vi "参数设置页.vi"() -> ()   [LabVIEW 2016, in "斯坦道通用流路CODmn.lvlib"]
uses:
  <vilib>/Plasmionique/MB Master/MB_Master/MB_Master.lvclass
  <vilib>/ptbypt/NI_PtbyPt.lvlib
panel:
  in  "手动模式":bool caption="手动模式(hd)"
  in  "简易流程周期设置":cluster{"switch button":bool, "设置按钮":bool}
  out "连接状态":bool
  in  "标样核查自动补测":bool caption="通讯连接"
  in  "跨度核查自动补测":bool caption="通讯连接"
  in  "零点核查自动补测":bool caption="通讯连接"
  in  "标样核查标液偏差":dbl caption="标样核查标液偏差："
  in  "跨度核查标液偏差":dbl caption="跨度核查标液偏差："
  in  "零点核查标液偏差":dbl caption="零点核查标液偏差："
  out "低量程上限":dbl caption="低量程上限："
  in  "简易流程路径":path=path "data/流程.xml"
  out "数据刷新时间":string
  in  "通讯连接":bool=TRUE
  out "MB table":enum32{"Serial", "TCP"}(tab)
  in  "请选择串口:":refnum<visa-resource-name>
  in  "IP":string="127.0.0.1"
  in  "PORT":string="1001"
  in  "通信方式选择":enum16{"串口", "TCP"}(ring)
  in  "盐度自动补偿：":bool
  out "盐度补偿值":dbl caption="盐度补偿值："
  in  "刷新":bool
  in  "测量模式":T1(ring)
  in  "参数下拉列表":u16(ring)
  in  "量程下拉列表":enum16{"低量程", "高量程"}(ring)
  in  "测试流程路径":path=path "data/流程.xml"
  in  "标样核查量程模式":T2 caption="标样核查："
  in  "加标回收量程模式":T2 caption="加标回收："
  in  "跨度核查量程模式":T2 caption="跨度核查："
  in  "零点核查量程模式":T2 caption="零点核查："
  in  "水样测试量程模式":T2 caption="水样测试："
  out "稀释度":dbl caption="稀释度："
  out "阈值（高->低）":dbl caption="阈值（高->低）："
  out "阈值（低->高）":dbl caption="阈值（低->高）："
  out "量程下限":dbl caption="量程下限："
  out "高量程上限":dbl caption="高量程上限："
  out "检出限":dbl caption="检出限："
  out "曲线截距":dbl caption="曲线截距：" format="%#.6f"
  out "曲线斜率":dbl caption="曲线斜率：" format="%#.6f"
  out "二次多项式系数":dbl caption="二次多项式系数：" format="%#.6f"
  out "消解时长":dbl caption="消解时长："
  out "消解温度":dbl caption="消解温度："
  out "测量精度":u16 caption="测量精度："
  in  "标样核查标液浓度":dbl caption="标样核查标液浓度："
  in  "跨度核查标液浓度":dbl caption="跨度核查标液浓度："
  in  "零点核查标液浓度":dbl caption="零点核查标液浓度："
  in  "跨度值":dbl caption="跨度值："
  # "日质控设置"
  # "关键参数"
  # "连接设置"
  # "mg/L"
  # "mg/L"
  # "mg/L"
  # "mg/L"
  # "±"
  # "%"
  # "%"
  # "流程设置"
  # "简易流程周期设置"
  # "自动测试量程设置"
  # "设置："
  # "mg/L"
  # "ppt"
  # "mg/L"
  # "mg/L"
  # "mg/L"
  # "mg/L"
  # "mg/L"
  # "min"
  # "℃"
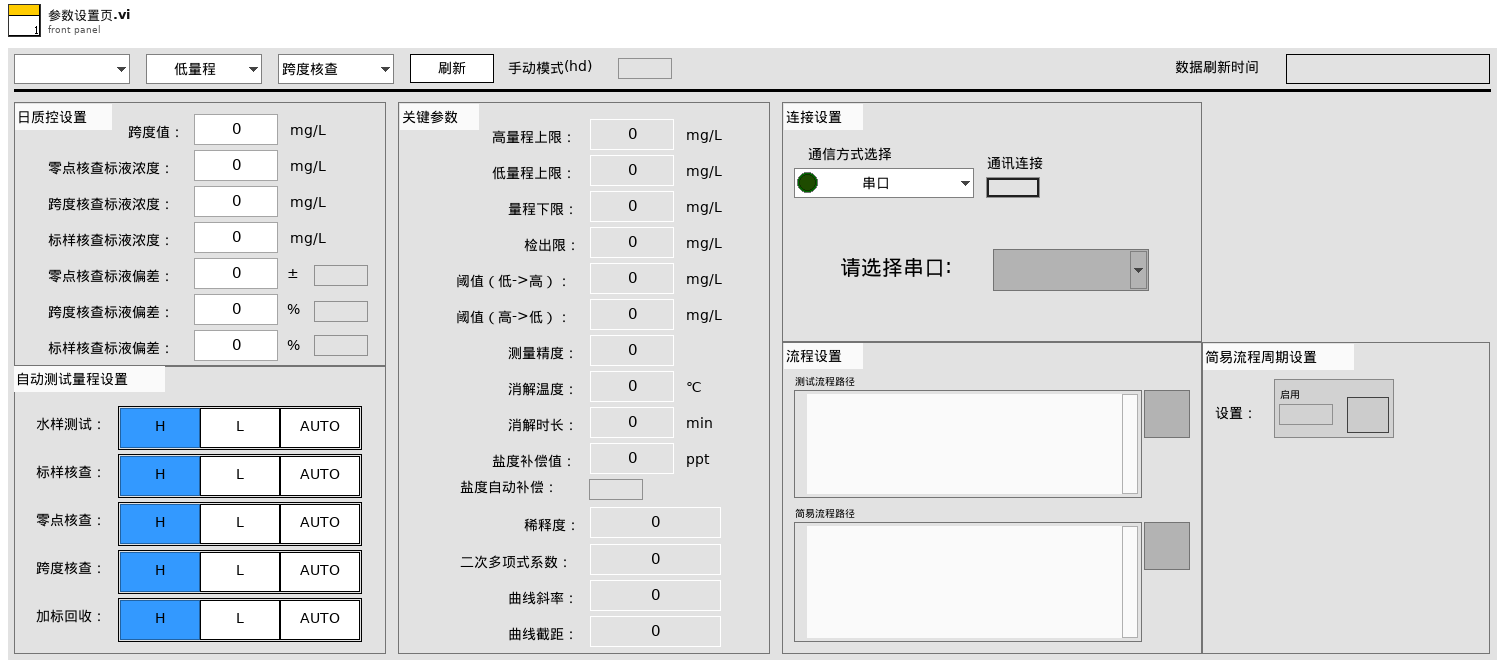
[diagram p1: front panel]
types:
  T1 = enum16{"跨度核查", "水样测量", "零点核查", "标样核查", "加标回收", "平行样测试", "空白校准", "标样校准", "空白测试"}
  T2 = typedef "斯坦道通用流路CODmn.lvlib/量程模式.ctl" = enum32{"H", "L", "AUTO"}
  T3 = typedef "Cleaning cycle.lvclass/周期项.ctl" = cluster{"时":i32, "分":i32, "频次":string, "id":i32, "参数":string, "simpleflowid":i32, "简易流程名称":string}
  T4 = cluster{"系统时间":timestamp, "工作状态":u16, "测量模式":enum16{"待机", "连续模式", "周期模式", "定点模式", "受控模式", "手动模式"}, "告警代码":u16, "故障代码":u16, "日志代码":u16, "软件版本":u16, "F0":sgl, "F1":sgl, "F2":sgl, "F3":sgl, "T":sgl, "H":sgl, "id":u16, "flowid":u16, "量程":u16, "总磷控温温度1":sgl, "营养盐控温温度2":sgl, "ADC":sgl, "结果值":sgl, "运行时间":u16, "步骤详情":string, "步骤流程":string}
  T5 = typedef "LVStringsAndValuesArrayTypeDef_U16.ctl" = cluster{"String":string, "Value":u16}[]
  T6 = enum8{"Enabled", "Disabled", "Disabled and Grayed Out"}
  T7 = cluster{"测量精度":u16, "检出限":dbl, "上限":dbl, "下限":dbl, "阈值（低->高）":dbl, "阈值（高->低）":dbl, "稀释度":dbl}
  T8 = typedef "操作日志字段定义.ctl" = cluster{"时间":timestamp, "参数":string, "日志信息":string, "流程参数":string}
  T9 = typedef "SingleStepTestV3.lvlib/SingleStepTestV3.lvclass/仪器版本.ctl" = enum16{"V3.1版", "V4版", "V3版", "V4.2版"}
  T10 = typedef "斯坦道通用流路CODmn.lvlib/V3.1版外设参数.ctl" = cluster{"泵类型":u8, "进样速度":u32, "出样速度":u32, "泵阀量":u8, "阀方向":u8, "光谱仪类型":u8, "光谱采样次数":u8, "氙灯次数":u8, "B":u16, "C":u16, "D":u16, "E":u16, "B_COD":u16, "C_COD":u16, "D_COD":u16, "E_COD":u16, "G":u16, "M":u16, "N":u16, "氨氮注射泵控温下限":sgl, "氨氮注射泵控温上限":sgl, "总氮注射泵控温下限":sgl, "总氮注射泵控温上限":sgl, "消解温度下限":sgl, "消解温度上限":sgl, "加热10s限值":sgl, "KP":sgl, "KI":sgl, "KD":sgl, "高温高压阀开阀温度":sgl, "总氮x公式0":u8, "总氮x公式1":sgl, "总氮x公式2":sgl, "总磷浊度稀释系数":sgl, "总磷浊度补偿权重1":sgl, "总磷浊度补偿权重2":sgl, "盐度系数":sgl, "氨氮补偿系数1":sgl, "氨氮补偿系数2":sgl}
  T11 = typedef "斯坦道通用流路CODmn.lvlib/V4版外设参数.ctl" = cluster{"泵类型":u8, "注射泵正常速度":u32, "注射泵慢速":u32, "阀型号":u8, "res":u8, "光谱仪类型":u8, "光谱采样次数":u8, "氙灯次数":u8, "B":u16, "C":u16, "D":u16, "E":u16, "B_COD":u16, "C_COD":u16, "D_COD":u16, "E_COD":u16, "G":u16, "M":u16, "N":u16, "降温下限":sgl, "降温上限":sgl, "恒温温度下限":sgl, "恒温温度上限":sgl, "消解温度下限":sgl, "消解温度上限":sgl, "加热10s限值":sgl, "KP":sgl, "KI":sgl, "KD":sgl, "高温高压阀开阀温度":sgl, "总氮x公式0":u8, "总氮x公式1":sgl, "总氮x公式2":sgl, "总磷浊度稀释系数":sgl, "总磷浊度补偿权重1":sgl, "总磷浊度补偿权重2":sgl, "盐度系数":sgl, "氨氮补偿系数1":sgl, "氨氮补偿系数2":sgl, "缺试剂传感器阈值":u16}
  T12 = typedef "斯坦道通用流路CODmn.lvlib/V4.2版外设参数.ctl" = cluster{"工作模式":u16, "泵类型":u16, "阀型号":u16, "注射泵进样速度":u16, "注射泵出样速度":u16, "注射泵滴定速度":u16, "res":u16, "注射泵慢速":u16, "光谱仪类型":u16, "光谱采样次数":u16, "氙灯次数":u16, "B":u16, "C":u16, "D":u16, "E":u16, "B_COD":u16, "C_COD":u16, "D_COD":u16, "E_COD":u16, "G":u16, "M":u16, "N":u16, "温度校准参数":sgl, "降温温度":sgl, "恒温温度":sgl, "消解温度":sgl, "高温高压阀开阀温度":sgl, "加热超时时间":sgl, "KP":sgl, "KI":sgl, "KD":sgl, "消解PID积分上限":sgl, "恒温PID积分上限":sgl, "PID积分下限":sgl, "缺试剂传感器阈值":u16, "滴定延时":u16, "滴定斜率阈值":sgl, "总氮x公式0":u16, "总氮x公式1":sgl, "总氮x公式2":sgl, "总磷浊度稀释系数":sgl, "总磷浊度补偿权重1":sgl, "总磷浊度补偿权重2":sgl, "盐度系数":sgl, "氨氮补偿系数1":sgl, "氨氮补偿系数2":sgl}
  T13 = typedef "斯坦道通用流路CODmn.lvlib/V3版外设参数.ctl" = cluster{"泵类型":u8, "进样速度":u32, "出样速度":u32, "泵阀量":u8, "光谱仪类型":u8, "光谱采样次数":u8, "氙灯次数":u8, "B":u16, "C":u16, "D":u16, "E":u16, "B_COD":u16, "C_COD":u16, "D_COD":u16, "E_COD":u16, "G":u16, "M":u16, "N":u16, "氨氮注射泵控温下限":sgl, "氨氮注射泵控温上限":sgl, "总氮注射泵控温下限":sgl, "总氮注射泵控温上限":sgl, "消解温度下限":sgl, "消解温度上限":sgl, "加热10s限值":sgl, "高温高压阀开阀温度":sgl, "总氮x公式0":u8, "总氮x公式1":sgl, "总氮x公式2":sgl, "总磷浊度稀释系数":sgl, "总磷浊度补偿权重1":sgl, "总磷浊度补偿权重2":sgl, "盐度系数":sgl, "氨氮补偿系数1":sgl, "氨氮补偿系数2":sgl}
  T14 = cluster{"水样测试量程模式":T2, "零点核查量程模式":T2, "跨度核查量程模式":T2, "加标回收量程模式":T2, "标样核查量程模式":T2}
  T15 = cluster{"总磷":dbl, "总氮":dbl, "氨氮":dbl, "磷酸盐":dbl, "硝氮":dbl, "亚硝氮":dbl, "硅酸盐":dbl, "硫化物":dbl, "COD":dbl, "氟化物":dbl, "CODMn":dbl}
  T16 = cluster{"总磷跨度值":dbl, "总磷零点标准液浓度":dbl, "总磷跨度标准液浓度":dbl, "总磷标准液标准浓度":dbl, "总氮跨度值":dbl, "总氮零点标准液浓度":dbl, "总氮跨度标准液浓度":dbl, "总氮标准液标准浓度":dbl, "COD跨度值":dbl, "COD零点标准液浓度":dbl, "COD跨度标准液浓度":dbl, "COD标准液标准浓度":dbl, "氨氮跨度值":dbl, "氨氮零点标准液浓度":dbl, "氨氮跨度标准液浓度":dbl, "氨氮标准液标准浓度":dbl, "磷酸盐跨度值":dbl, "磷酸盐零点标准液浓度":dbl, "磷酸盐跨度标准液浓度":dbl, "磷酸盐标准液标准浓度":dbl, "硝氮跨度值":dbl, "硝氮零点标准液浓度":dbl, "硝氮跨度标准液浓度":dbl, "硝氮标准液标准浓度":dbl, "亚硝氮跨度值":dbl, "亚硝氮零点标准液浓度":dbl, "亚硝氮跨度标准液浓度":dbl, "亚硝氮标准液标准浓度":dbl, "硫化物跨度值":dbl, "硫化物零点标准液浓度":dbl, "硫化物跨度标准液浓度":dbl, "硫化物标准液标准浓度":dbl, "硅酸盐跨度值":dbl, "硅酸盐零点标准液浓度":dbl, "硅酸盐跨度标准液浓度":dbl, "硅酸盐标准液标准浓度":dbl, "总磷零点标准液偏差":dbl, "总磷跨度标准液偏差":dbl, "总磷标准液标准偏差":dbl, "总氮零点标准液偏差":dbl, "总氮跨度标准液偏差":dbl, "总氮标准液标准偏差":dbl, "COD零点标准液偏差":dbl, "COD跨度标准液偏差":dbl, "COD标准液标准偏差":dbl, "氨氮零点标准液偏差":dbl, "氨氮跨度标准液偏差":dbl, "氨氮标准液标准偏差":dbl, "磷酸盐零点标准液偏差":dbl, "磷酸盐跨度标准液偏差":dbl, "磷酸盐标准液标准偏差":dbl, "硝氮零点标准液偏差":dbl, "硝氮跨度标准液偏差":dbl, "硝氮标准液标准偏差":dbl, "亚硝氮零点标准液偏差":dbl, "亚硝氮跨度标准液偏差":dbl, "亚硝氮标准液标准偏差":dbl, "硫化物零点标准液偏差":dbl, "硫化物跨度标准液偏差":dbl, "硫化物标准液标准偏差":dbl, "硅酸盐零点标准液偏差":dbl, "硅酸盐跨度标准液偏差":dbl, "硅酸盐标准液标准偏差":dbl, "氟化物跨度值":dbl, "氟化物零点标准液浓度":dbl, "氟化物跨度标准液浓度":dbl, "氟化物标准液标准浓度":dbl, "氟化物零点标准液偏差":dbl, "氟化物跨度标准液偏差":dbl, "氟化物标准液标准偏差":dbl, "CODMn跨度值":dbl, "CODMn零点标准液浓度":dbl, "CODMn跨度标准液浓度":dbl, "CODMn标准液标准浓度":dbl, "CODMn零点标准液偏差":dbl, "CODMn跨度标准液偏差":dbl, "CODMn标准液标准偏差":dbl}
  T17 = cluster{"水样测试量程模式":enum16{"H", "L", "AUTO"}, "空白核查量程模式":enum16{"H", "L", "AUTO"}, "跨度核查量程模式":enum16{"H", "L", "AUTO"}, "加标回收量程模式":enum16{"H", "L", "AUTO"}, "标样核查量程模式":enum16{"H", "L", "AUTO"}}
  T18 = cluster{"水样测试量程模式":u16, "空白核查量程模式":u16, "跨度核查量程模式":u16, "加标回收量程模式":u16, "标样核查量程模式":u16}
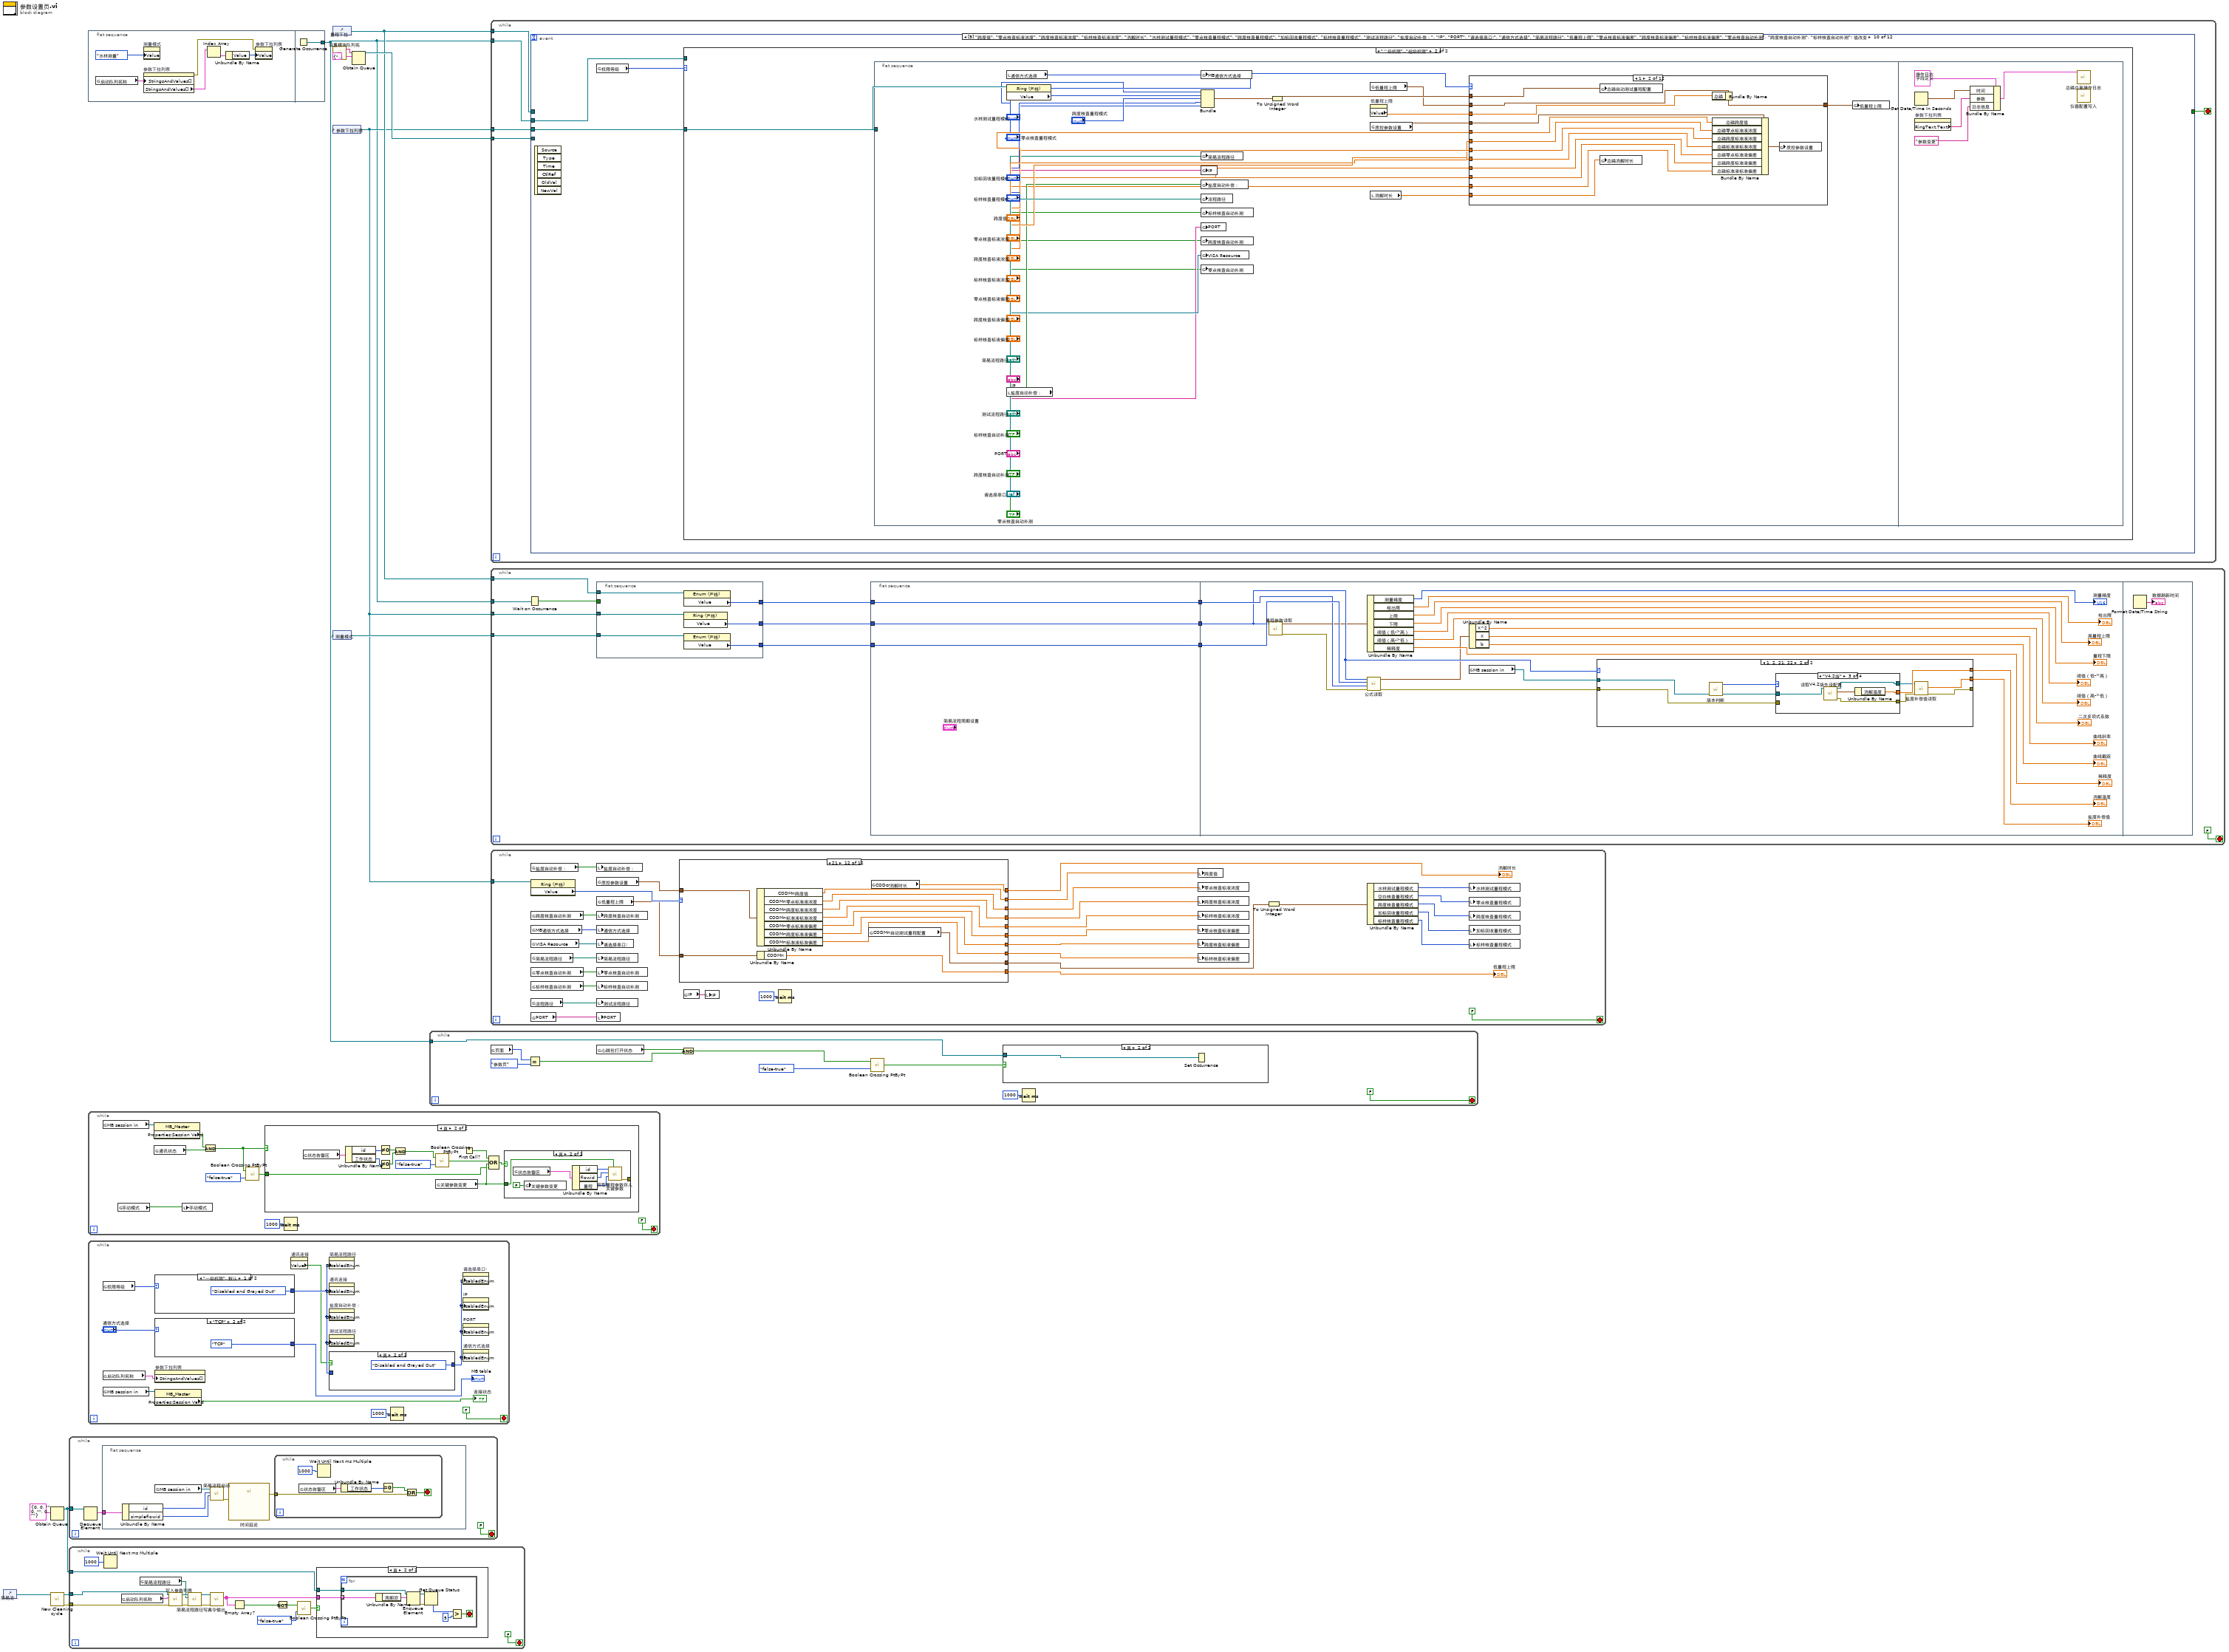
[diagram p0: block diagram]
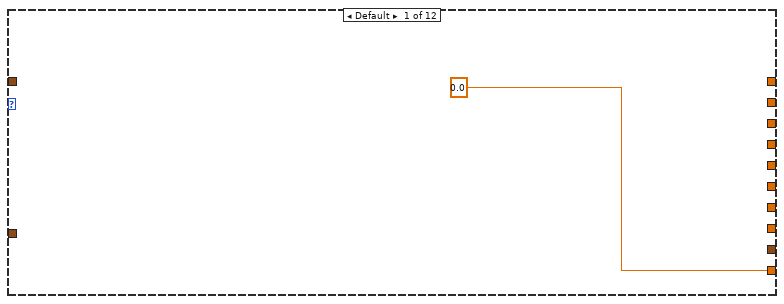
[diagram p6: hidden frame]
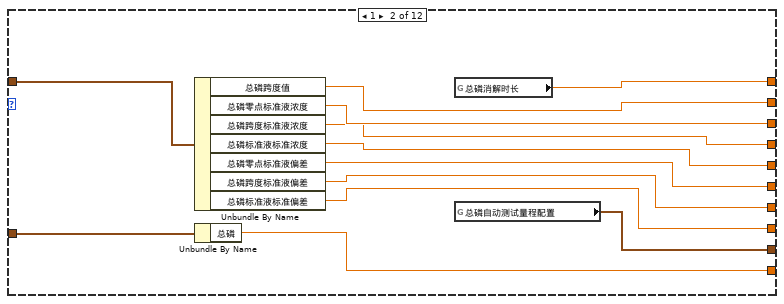
[diagram p7: hidden frame]
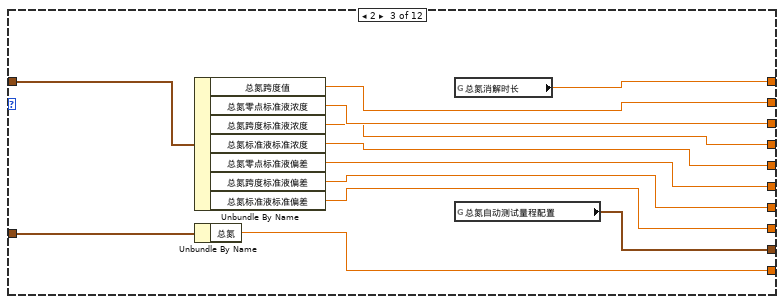
[diagram p8: hidden frame]
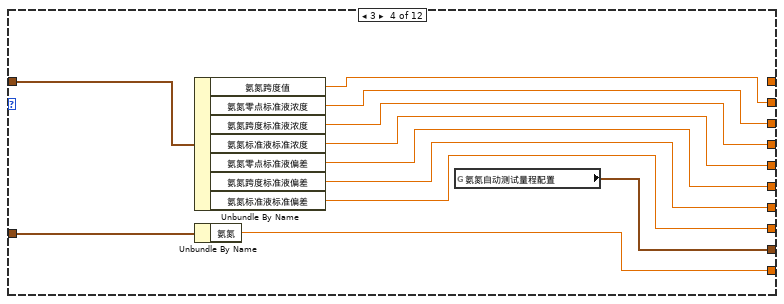
[diagram p9: hidden frame]
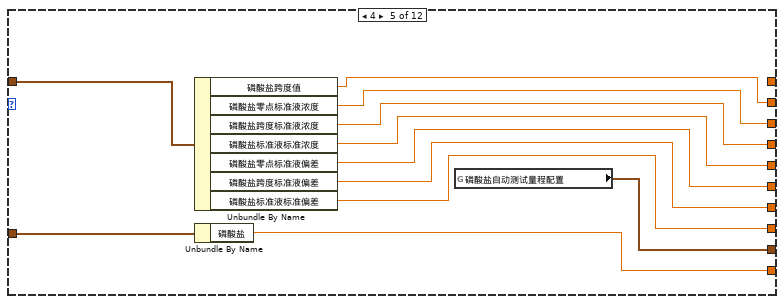
[diagram p10: hidden frame]
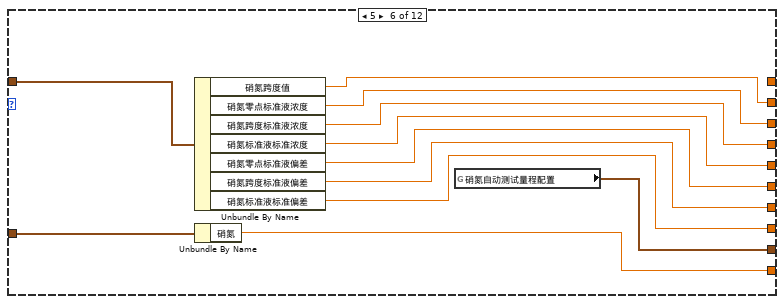
[diagram p11: hidden frame]
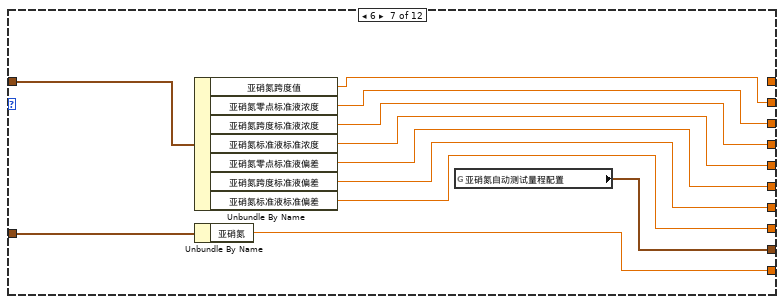
[diagram p12: hidden frame]
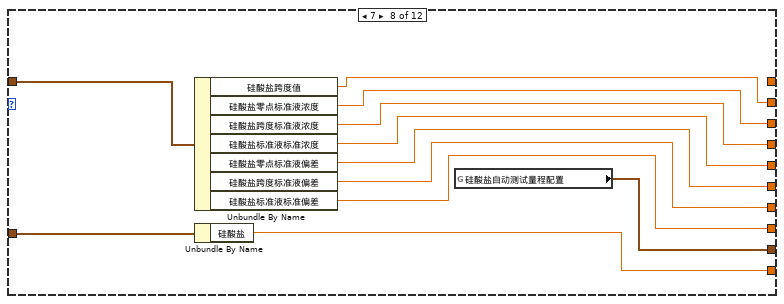
[diagram p13: hidden frame]
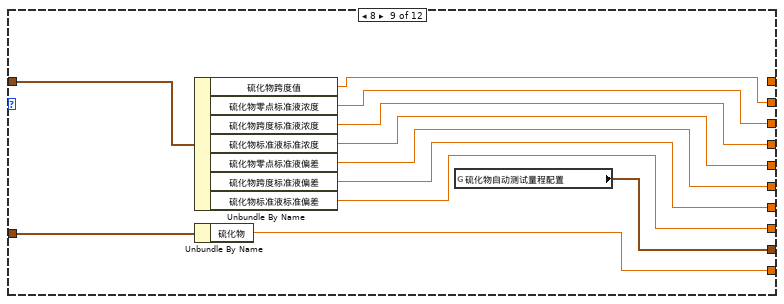
[diagram p14: hidden frame]
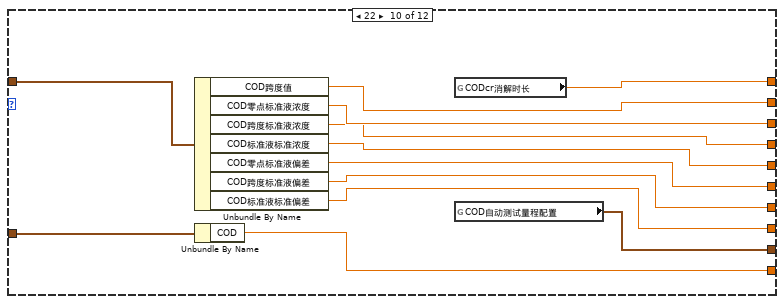
[diagram p15: hidden frame]
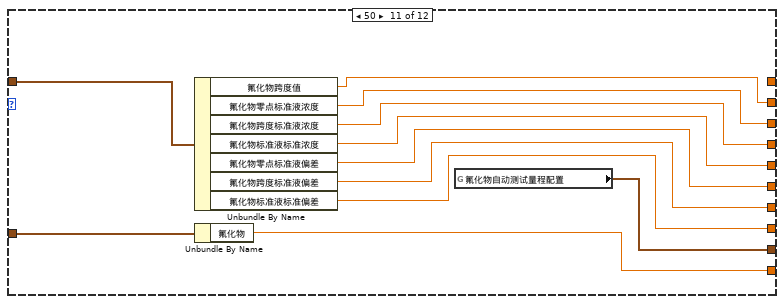
[diagram p16: hidden frame]
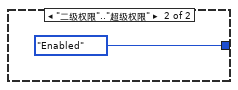
[diagram p17: hidden frame]
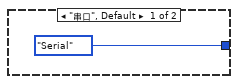
[diagram p18: hidden frame]
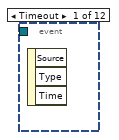
[diagram p20: hidden frame]
diagram:
  n1 = control-ref of="简易流程周期设置"() -> (w3:refnum<vi>)
  n2 = Obtain Queue(element data type=T3 {"时"=0, "分"=0, "频次"="", "id"=0, "参数"="", "simpleflowid"=0, "简易流程名称"=""} ("周期项")) -> (queue out=w1:refnum<queue>)  [unwired: 4 in, 2 out]
  n3 = call "New Cleaning cycle.vi"("Reference"=w3) -> ("error out"=w4:errorcluster, "Cleaningcycle out"=w5:refnum<class "Cleaning cycle.lvclass">)  [unwired: 9 in]
  n4 = while {
    tunnel: w1 -> [w15]
    stop <- FALSE stop-if-true
    n5 = Dequeue Element(queue=w15) -> (element=w14:T3)  [unwired: 2 in, 3 out]
    n6 = flat-sequence {
      tunnel: w14 -> [w20]
      frame #0 {
        n7 = Unbundle By Name(w20) -> ("id"=w18:i32, "simpleflowid"=w19:i32)
        n8 = global read "VAR总磷总氮全局变量.vi" "MB session in"() -> (w21:refnum<class "MB_Master.lvclass">)
        n9 = call "简易流程启动.vi"("简易流程"=w19, "参数Id"=w18, "MB session in"=w21) -> ("error out"=w17:errorcluster)  [unwired: 7 in, 1 out]
        n10 = call "时间延迟"("error in (no error)"=w17) -> ("error out"=w16:errorcluster)  [unwired: 10 in]
        n11 = while {
          tunnel: w16 -> [w23]
          stop <- w22 stop-if-true
          n12 = global read "VAR总磷总氮全局变量.vi" "状态告警区"() -> (w26:T4)
          n13 = Wait Until Next ms Multiple(millisecond multiple=u32 1000 ("毫秒倍数")) -> ()  [unwired: 1 out]
          n14 = Unbundle By Name(w26) -> ("工作状态"=w25:u16)
          n15 = Equal To 0?(x=w25) -> (x = 0?=w24:bool)
          n16 = Or(x=w24, y=w23) -> (x .or. y?=w22:bool)
        }
      }
    }
  }
  n17 = while {
    tunnel: w5 -> [w43]
    tunnel: w4 -> [w42]
    tunnel: w1 -> [w29]
    stop <- FALSE stop-if-true
    n18 = Wait Until Next ms Multiple(millisecond multiple=u32 1000 ("毫秒倍数")) -> ()  [unwired: 1 out]
    n19 = global read "model config var.vi" "启动队列名称"() -> (w39:cluster{"String":string, "Value":u16}[])
    n20 = global read "总磷总氮断电保存全局变量.vi" "简易流程路径"() -> (w38:path)
    n21 = call "写入参数列表.vi"("error in (no error)"=w42, "参数列表"=w39, "Cleaningcycle 输入"=w43) -> ("error out"=w41:errorcluster, "Cleaningcycle 输出"=w40:refnum<class "Cleaning cycle.lvclass">)  [unwired: 7 in]
    n22 = call "简易流程路径写入.vi"("error in (no error)"=w41, "简易流程路径"=w38, "Cleaningcycle 输入"=w40) -> ("error out"=w36:errorcluster, "Cleaningcycle 输出"=w37:refnum<class "Cleaning cycle.lvclass">)  [unwired: 7 in]
    n23 = call "命令输出.vi"("error in (no error)"=w36, "Cleaningcycle 输入"=w37) -> ("命令"=w31:cluster{"触发":bool, "周期项":T3}[])  [unwired: 7 in, 2 out]
    n24 = Empty Array?(array=w31) -> (empty?=w35:bool)
    n25 = Not(x=w35) -> (.not. x?=w34:bool)
    n26 = call <vilib>:"Boolean Crossing PtByPt.vi"("direction"=enum16{"either", "false-true", "true-false"}."false-true", "input"=w34) -> ("crossing"=w32:bool)  [unwired: 1 in]
    n27 = case shown="真" w32 {
      tunnel: w31 -> [_ w45]
      tunnel: w29 -> [_ w44]
      frame False {
      }
      frame True {
        n28 = for {
          tunnel: w45 -> [w53] mode=indexing
          tunnel: w44 -> [w51]
          stop <- w46 stop-if-true
          n29 = Unbundle By Name(w53) -> ("周期项"=w52:T3)
          n30 = Enqueue Element(queue=w51, element=w52) -> (queue out=w50:refnum<queue>, error out=w49:errorcluster)  [unwired: 2 in, 1 out]
          n31 = Get Queue Status(queue=w50, error in (no error)=w49) -> (# elements in queue=w48:i32)  [unwired: 1 in, 7 out]
          n32 = Greater?(x=w48, y=5) -> (0:w46:bool)
        }
      }
    }
  }
  n33 = flat-sequence {
    tunnel: [w60] -> w6
    frame #0 {
      n34 = global read "model config var.vi" "启动队列名称"() -> (w55:cluster{"String":string, "Value":u16}[])
      n35 = property on="测量模式" class="Enum (严格)"("Value"=T1."水样测量" ("测量模式")) -> ()  [unwired: 2 in, 2 out]
      n36 = property on="参数下拉列表" class="Ring (严格)"("StringsAndValues[]"=w55) -> (error out=w58:errorcluster, "StringsAndValues[]"=w56:T5)  [unwired: 2 in, 1 out]
      n37 = Index Array(array=w56) -> (element=w57:cluster{"String":string, "Value":u16})  [unwired: 1 in]
      n38 = Unbundle By Name(w57) -> ("Value"=w59:u16)
      n39 = property on="参数下拉列表" class="Ring (严格)"(error in=w58, "Value"=w59) -> ()  [unwired: 1 in, 2 out]
    }
    frame #1 {
      n40 = Generate Occurrence() -> (w60:refnum<k4>)
    }
  }
  n41 = while {
    stop <- FALSE stop-if-true
    n42 = global read "VAR总磷总氮全局变量.vi" "MB session in"() -> (w66:refnum<class "MB_Master.lvclass">)
    n43 = global read "VAR总磷总氮全局变量.vi" "手动模式"() -> (w61:bool)
    n44 = property class="MB_Master"(reference=w66) -> ("Properties:Session Valid"=w65:bool)  [unwired: 1 in, 2 out]
    n45 = global read "VAR总磷总氮全局变量.vi" "通讯状态"() -> (w68:bool)
    n46 = local write "手动模式"(w61) -> ()
    n47 = And(x=w65, y=w68) -> (x .and. y?=w63:bool)
    n48 = call <vilib>:"Boolean Crossing PtByPt.vi"("direction"=enum16{"either", "false-true", "true-false"}."false-true", "input"=w63) -> ("crossing"=w62:bool)  [unwired: 1 in]
    n49 = case shown="真" w63 {
      tunnel: w62 -> [_ w71]
      frame False {
      }
      frame True {
        n50 = global read "VAR总磷总氮全局变量.vi" "状态告警区"() -> (w81:T4)
        n51 = Unbundle By Name(w81) -> ("id"=w75:u16, "工作状态"=w80:u16)
        n52 = Not Equal To 0?(x=w75) -> (x != 0?=w76:bool)
        n53 = Not Equal To 0?(x=w80) -> (x != 0?=w77:bool)
        n54 = And(x=w76, y=w77) -> (x .and. y?=w78:bool)
        n55 = call <vilib>:"Boolean Crossing PtByPt.vi"("direction"=enum16{"either", "false-true", "true-false"}."false-true", "input"=w78) -> ("crossing"=w74:bool)  [unwired: 1 in]
        n56 = global read "VAR总磷总氮全局变量.vi" "关键参数变更"() -> (w72:bool)
        n57 = First Call?() -> (First Call?: T/F=w70:bool)
        n58 = Compound Arithmetic op=OR ("复合运算")(w70, w74, w72, w71) -> (w73:bool)
        n59 = case shown="真" w73 {
          tunnel: [_ w88] -> _
          tunnel: w72 -> [_ w83]
          frame False {
          }
          frame True {
            n60 = global read "VAR总磷总氮全局变量.vi" "状态告警区"() -> (w87:T4)
            n61 = global write "VAR总磷总氮全局变量.vi" "关键参数变更"(FALSE ("关键参数变更")) -> ()
            n62 = Unbundle By Name(w87) -> ("id"=w86:u16, "flowid"=w85:u16, "量程"=w84:u16)
            n63 = call "获取量程参数存入关键参数.vi"("关键参数变更"=w83, "量程"=w84, "flowid"=w85, "id"=w86) -> ("error out"=w88:errorcluster)  [unwired: 7 in]
          }
        }
      }
    }
    n64 = Wait (ms)(milliseconds to wait=u32 1000 ("等待时间（毫秒）")) -> ()  [unwired: 1 out]
  }
  n65 = while {
    stop <- FALSE stop-if-true
    n66 = global read "VAR总磷总氮全局变量.vi" "权限等级"() -> (w93:enum16{"一级权限", "二级权限", "三级权限", "超级权限"})
    n67 = global read "model config var.vi" "启动队列名称"() -> (w91:cluster{"String":string, "Value":u16}[])
    n68 = global read "VAR总磷总氮全局变量.vi" "MB session in"() -> (w98:refnum<class "MB_Master.lvclass">)
    n69 = case shown="\"一级权限\", 默认" w93 {
      tunnel: [T6."Disabled and Grayed Out" ("禁用") T6."Enabled" ("禁用")] -> w92
      frame "一级权限", Default {
      }
      frame "二级权限".."超级权限" {
      }
    }
    n70 = case shown="\"TCP\"" "通信方式选择" {
      tunnel: [enum32{"Serial", "TCP"}."Serial" ("MB table") enum32{"Serial", "TCP"}."TCP" ("MB table")] -> w95
      frame "串口", Default {
      }
      frame "TCP" {
      }
    }
    "MB table" <- w95
    n71 = property on="参数下拉列表" class="Ring (严格)"("StringsAndValues[]"=w91) -> ()  [unwired: 2 in, 2 out]
    n72 = property class="MB_Master"(reference=w98) -> ("Properties:Session Valid"=→"连接状态":bool)  [unwired: 1 in, 2 out]
    n73 = property on="通讯连接" class="Bool (严格)"() -> ("Value"=w89:bool)  [unwired: 2 in, 2 out]
    n74 = property on="简易流程路径" class="Path"("DisabledEnum"=w92) -> ()  [unwired: 2 in, 2 out]
    n75 = property on="通讯连接" class="Bool (严格)"("DisabledEnum"=w92) -> ()  [unwired: 2 in, 2 out]
    n76 = property on="盐度自动补偿：" class="Bool (严格)"("DisabledEnum"=w92) -> ()  [unwired: 2 in, 2 out]
    n77 = property on="测试流程路径" class="Path"("DisabledEnum"=w92) -> ()  [unwired: 2 in, 2 out]
    n78 = case shown="真" w89 {
      tunnel: [w104 T6."Disabled and Grayed Out" ("禁用")] -> w96
      tunnel: w92 -> [w104 _]
      frame False {
      }
      frame True {
      }
    }
    n79 = Wait (ms)(milliseconds to wait=u32 1000 ("等待时间（毫秒）")) -> ()  [unwired: 1 out]
    n80 = property on="请选择串口:" class="VISAName"("DisabledEnum"=w96) -> ()  [unwired: 2 in, 2 out]
    n81 = property on="IP" class="Str"("DisabledEnum"=w96) -> ()  [unwired: 2 in, 2 out]
    n82 = property on="PORT" class="Str"("DisabledEnum"=w96) -> ()  [unwired: 2 in, 2 out]
    n83 = property on="通信方式选择" class="Enum (严格)"("DisabledEnum"=w96) -> ()  [unwired: 2 in, 2 out]
  }
  n84 = control-ref of="量程下拉列表"() -> (w8:refnum<vi>)
  n85 = call "设置模块队列名.vi"() -> ("Msg"=w11:string)  [unwired: 5 in]
  n86 = control-ref of="参数下拉列表"() -> (w7:refnum<vi>)
  n87 = control-ref of="测量模式"() -> (w9:refnum<vi>)
  n88 = Obtain Queue(name (unnamed)=w11, element data type=cluster{"命令":string, "data":variant} {"命令"="", "data"=variant}) -> (queue out=w10:refnum<queue>)  [unwired: 3 in, 2 out]
  n89 = while {
    tunnel: w6 -> [w112]
    stop <- FALSE stop-if-true
    n90 = global read "VAR总磷总氮全局变量.vi" "页面"() -> (w114:enum16{"主页", "参数页", "校准页"})
    n91 = Equal?(x=w114, y=enum16{"主页", "参数页", "校准页"}."参数页" ("页面")) -> (x = y?=w113:bool)
    n92 = global read "VAR总磷总氮全局变量.vi" "心跳包打开状态"() -> (w108:bool)
    n93 = And(x=w108, y=w113) -> (x .and. y?=w109:bool)
    n94 = call <vilib>:"Boolean Crossing PtByPt.vi"("direction"=enum16{"either", "false-true", "true-false"}."false-true", "input"=w109) -> ("crossing"=w107:bool)  [unwired: 1 in]
    n95 = case shown="真" w107 {
      tunnel: w112 -> [_ w116]
      frame False {
      }
      frame True {
        n96 = Set Occurrence(w116) -> ()
      }
    }
    n97 = Wait (ms)(milliseconds to wait=u32 1000 ("等待时间（毫秒）")) -> ()  [unwired: 1 out]
  }
  n98 = while {
    tunnel: w6 -> [w120]
    tunnel: w7 -> [w119]
    tunnel: w10 -> [w118]
    tunnel: w8 -> [w117]
    stop <- w121 stop-if-true
    n99 = event shown="[9] \"跨度值\", \"零点核查标液浓度\", \"跨度核查标液浓度\", \"标样核查标液浓度\", \"消解时长\", \"水样测试量程模式\", \"零点核查量程模式\", \"跨度核查量程模式\", \"加标回收量程模式\", \"标样核查量程模式\", \"测试流程路径\", \"盐度自动补偿：\", \"IP\", \"PORT\", \"请选择串口:\", \"通信方式选择\", \"简易流程路径\", \"低量程上限\", \"零点核查标液偏差\", \"跨度核查标液偏差\", \"标样核查标液偏差\", \"零点核查自动补测\", \"跨度核查自动补测\", \"标样核查自动补测\": 值改变" {
      selector: _ -> [_ _ _ _ _ _ _ _ _ _ _ _]
      dyn-events: _ -> [_ _ _ _ _ _ _ _ _ _ _ _]
      timeout: _ -> [_ _ _ _ _ _ _ _ _ _ _ _]
      tunnel: [_ TRUE _ _ _ _ _ _ _ _ _ _] -> w121
      tunnel: w120 -> [_ _ w123 _ _ _ _ _ _ w202 _ _]
      tunnel: w119 -> [_ _ _ _ w142 _ _ _ _ w204 _ _]
      tunnel: w118 -> [_ _ _ _ _ _ _ _ _ _ w392 _]
      tunnel: w117 -> [_ _ _ _ _ _ _ _ _ _ _ _]
      event Timeout {
        n100 = event-data() -> ()  [unwired: 1 in, 3 out]
      }
      event Panel Close {
        n101 = event-data() -> ()  [unwired: 1 in, 4 out]
      }
      event "参数下拉列表", "量程下拉列表", "测量模式", "刷新": Value Change {
        n102 = event-data() -> ()  [unwired: 1 in, 6 out]
        n103 = Set Occurrence(w123) -> ()
      }
      event "跨度值", "零点核查标液浓度", "跨度核查标液浓度", "标样核查标液浓度", "消解温度", "消解时长", "检出限", "高量程上限", "量程下限", "阈值（低->高）", "阈值（高->低）", "稀释度", "低量程上限", "零点核查标液偏差", "跨度核查标液偏差", "标样核查标液偏差": Mouse Down {
        n104 = event-data() -> ("CtlRef"=w125:refnum<vi>)  [unwired: 1 in, 5 out]
        n105 = global read "VAR总磷总氮全局变量.vi" "权限等级"() -> (w124:enum16{"一级权限", "二级权限", "三级权限", "超级权限"})
        n106 = case shown="\"二级权限\"..\"超级权限\"" w124 {
          tunnel: w125 -> [_ w129]
          frame "一级权限", Default {
          }
          frame "二级权限".."超级权限" {
            n107 = property class="DigNum (严格)"(reference=w129) -> (reference out=w127:refnum<vi>, "Value"=w128:dbl)  [unwired: 1 in, 1 out]
            n108 = call "数字键盘.vi"("OldNumber"=w128) -> ("NewNumber"=w126:dbl)
            n109 = property class="DigNum (严格)"(reference=w127, "Val(Sgnl)"=w126) -> ()  [unwired: 1 in, 2 out]
          }
        }
      }
      event "测量精度", "检出限", "高量程上限", "量程下限", "阈值（低->高）", "阈值（高->低）", "稀释度": Value Change {
        n110 = event-data() -> ()  [unwired: 1 in, 6 out]
        n111 = local read "测量精度"() -> (w132:u16)
        n112 = local read "检出限"() -> (w136:dbl)
        n113 = local read "高量程上限"() -> (w138:dbl)
        n114 = local read "量程下限"() -> (w137:dbl)
        n115 = local read "阈值（低->高）"() -> (w135:dbl)
        n116 = local read "阈值（高->低）"() -> (w134:dbl)
        n117 = local read "稀释度"() -> (w133:dbl)
        n118 = property class="Ring (严格)"(reference=w142) -> ("Value"=w141:u16)  [unwired: 1 in, 2 out]
        n119 = Bundle By Name(cluster=T7 {"测量精度"=0, "检出限"=0.0, "上限"=0.0, "下限"=0.0, "阈值（低->高）"=0.0, "阈值（高->低）"=0.0, "稀释度"=0.0} ("量程参数写入"), "测量精度"=w132, "检出限"=w136, "上限"=w138, "下限"=w137, "阈值（低->高）"=w135, "阈值（高->低）"=w134, "稀释度"=w133) -> (w139:T7)
        n120 = call "量程参数写入.vi"("量程参数写入"=w139, "测量参数"=w141) -> ("error out"=w130:errorcluster)  [unwired: 8 in]
        n121 = case shown="无错误" w130 {
          tunnel: ["写入成功" "写入失败"] -> w131
          frame No Error {
            n122 = Get Date/Time In Seconds() -> (seconds since 1Jan1904=w145:timestamp)
            n123 = property on="参数下拉列表" class="Ring (严格)"() -> ("RingText.Text"=w143:string)  [unwired: 2 in, 2 out]
            n124 = Bundle By Name(cluster=T8 {"时间"=timestamp(0 s since 1904-01-01), "参数"="", "日志信息"="", "流程参数"=""} ("data in"), "时间"=w145, "参数"=w143, "日志信息"="关键参数变更") -> (w146:T8)
            n125 = call "总磷总氮操作日志.vi"("data in"=w146) -> ()  [unwired: 10 in, 1 out]
            n126 = global write "VAR总磷总氮全局变量.vi" "关键参数变更"(TRUE ("关键参数变更")) -> ()
          }
          frame Error {
          }
        }
        n127 = One Button Dialog(message=w131) -> ()  [unwired: 1 in, 1 out]
      }
      event "消解温度": Value Change {
        n128 = event-data() -> ("NewVal"=w152:dbl)  [unwired: 1 in, 5 out]
        n129 = global read "VAR总磷总氮全局变量.vi" "MB session in"() -> (w153:refnum<class "MB_Master.lvclass">)
        n130 = call "版本判断.vi"() -> ("仪器版本"=w154:T9)  [unwired: 11 in]
        n131 = case shown="\"V4.2版\"" w154 {
          tunnel: w153 -> [w162 w169 w176 w183]
          tunnel: w152 -> [w157 w165 w172 w179]
          tunnel: [w156 w163 w170 w177] -> w151
          frame "V3.1版", Default {
            n132 = call "读取V3.1外设配置.vi"("MB session in"=w162) -> ("error out"=w158:errorcluster, "外设配置"=w161:T10, "MB session out"=w160:refnum<class "MB_Master.lvclass">)  [unwired: 8 in]
            n133 = Bundle By Name(cluster=w161, "消解温度下限"=w157) -> (w159:T10)
            n134 = call "写入V3.1外设配置.vi"("error in (no error)"=w158, "外设配置"=w159, "MB session in"=w160) -> ("error out"=w156:errorcluster)  [unwired: 7 in, 1 out]
          }
          frame "V4版" {
            n135 = call "读取V4版外设配置.vi"("MB session in"=w169) -> ("error out"=w164:errorcluster, "外设配置"=w167:T11, "MB session out"=w168:refnum<class "MB_Master.lvclass">)  [unwired: 8 in]
            n136 = Bundle By Name(cluster=w167, "消解温度下限"=w165) -> (w166:T11)
            n137 = call "写入V4版外设配置.vi"("error in (no error)"=w164, "外设配置"=w166, "MB session in"=w168) -> ("error out"=w163:errorcluster)  [unwired: 7 in, 1 out]
          }
          frame "V4.2版" {
            n138 = call "读取V4.2版外设配置.vi"("MB session in"=w176) -> ("error out"=w171:errorcluster, "外设配置"=w174:T12, "MB session out"=w175:refnum<class "MB_Master.lvclass">)  [unwired: 8 in]
            n139 = Bundle By Name(cluster=w174, "消解温度"=w172) -> (w173:T12)
            n140 = call "写入V4.2版外设配置.vi"("error in (no error)"=w171, "外设配置"=w173, "MB session in"=w175) -> ("error out"=w170:errorcluster)  [unwired: 7 in, 1 out]
          }
          frame "V3版" {
            n141 = call "读取V3外设配置.vi"("MB session in"=w183) -> ("error out"=w178:errorcluster, "外设配置"=w181:T13, "MB session out"=w182:refnum<class "MB_Master.lvclass">)  [unwired: 8 in]
            n142 = Bundle By Name(cluster=w181, "消解温度下限"=w179) -> (w180:T13)
            n143 = call "写入V3外设配置.vi"("error in (no error)"=w178, "外设配置"=w180, "MB session in"=w182) -> ("error out"=w177:errorcluster)  [unwired: 7 in, 1 out]
          }
        }
        n144 = case shown="错误" w151 {
          tunnel: ["写入成功" "写入失败"] -> w155
          frame No Error {
          }
          frame Error {
          }
        }
        n145 = One Button Dialog(message=w155) -> ()  [unwired: 1 in, 1 out]
      }
      event "测量精度": Mouse Down {
        n146 = event-data() -> ("CtlRef"=w187:refnum<vi>)  [unwired: 1 in, 7 out]
        n147 = global read "VAR总磷总氮全局变量.vi" "权限等级"() -> (w186:enum16{"一级权限", "二级权限", "三级权限", "超级权限"})
        n148 = case shown="\"二级权限\"..\"超级权限\"" w186 {
          tunnel: w187 -> [_ w191]
          frame "一级权限", Default {
          }
          frame "二级权限".."超级权限" {
            n149 = property class="DigNum (严格)"(reference=w191) -> (reference out=w189:refnum<vi>, "Value"=w190:u16)  [unwired: 1 in, 1 out]
            n150 = call "数字键盘.vi"("OldNumber"=w190) -> ("NewNumber"=w188:dbl)
            n151 = property class="DigNum (严格)"(reference=w189, "Val(Sgnl)"=w188) -> ()  [unwired: 1 in, 2 out]
          }
        }
      }
      event "盐度补偿值": Mouse Down {
        n152 = event-data() -> ("CtlRef"=w193:refnum<vi>)  [unwired: 1 in, 3 out]
        n153 = global read "VAR总磷总氮全局变量.vi" "权限等级"() -> (w192:enum16{"一级权限", "二级权限", "三级权限", "超级权限"})
        n154 = case shown="\"二级权限\"..\"超级权限\"" w192 {
          tunnel: w193 -> [_ w195]
          frame "一级权限", Default {
          }
          frame "二级权限".."超级权限" {
            n155 = case shown="假" "盐度自动补偿：" {
              tunnel: w195 -> [w199 _]
              frame False {
                n156 = property class="DigNum (严格)"(reference=w199) -> (reference out=w197:refnum<vi>, "Value"=w198:dbl)  [unwired: 1 in, 1 out]
                n157 = call "数字键盘.vi"("OldNumber"=w198) -> ("NewNumber"=w196:dbl)
                n158 = property class="DigNum (严格)"(reference=w197, "Val(Sgnl)"=w196) -> ()  [unwired: 1 in, 2 out]
              }
              frame True {
              }
            }
          }
        }
      }
      event "盐度补偿值": Value Change {
        n159 = event-data() -> ("NewVal"=w200:dbl)  [unwired: 1 in, 5 out]
        n160 = global read "VAR总磷总氮全局变量.vi" "MB session in"() -> (w201:refnum<class "MB_Master.lvclass">)
        n161 = call "盐度补偿值写入.vi"("盐度补偿值"=w200, "MB session in"=w201) -> ()  [unwired: 8 in, 2 out]
      }
      event "跨度值", "零点核查标液浓度", "跨度核查标液浓度", "标样核查标液浓度", "消解时长", "测试流程路径", "盐度自动补偿：", "IP", "PORT", "请选择串口:", "通信方式选择", "简易流程路径", "低量程上限", "零点核查标液偏差", "跨度核查标液偏差", "标样核查标液偏差", "零点核查自动补测", "跨度核查自动补测", "标样核查自动补测": Value Change {
        n162 = event-data() -> ()  [unwired: 1 in, 6 out]
        n163 = global read "VAR总磷总氮全局变量.vi" "权限等级"() -> (w203:enum16{"一级权限", "二级权限", "三级权限", "超级权限"})
        n164 = case shown="\"二级权限\"..\"超级权限\"" w203 {
          tunnel: w204 -> [_ w206]
          tunnel: w202 -> [w205 _]
          frame "一级权限", Default {
            n165 = Set Occurrence(w205) -> ()
          }
          frame "二级权限".."超级权限" {
            n166 = flat-sequence {
              tunnel: w206 -> [w236]
              frame #0 {
                n167 = local read "通信方式选择"() -> (w218:enum16{"串口", "TCP"})
                n168 = property class="Ring (严格)"(reference=w236) -> ("Value"=w235:u16)  [unwired: 1 in, 2 out]
                n169 = local read "盐度自动补偿："() -> (w222:bool)
                n170 = global write "总磷总氮断电保存全局变量.vi" "MB通信方式选择"(w218) -> ()
                n171 = Bundle("水样测试量程模式"="水样测试量程模式", "零点核查量程模式"="零点核查量程模式", "跨度核查量程模式"="跨度核查量程模式", "加标回收量程模式"="加标回收量程模式", "标样核查量程模式"="标样核查量程模式") -> (w224:T14)  [unwired: 1 in]
                n172 = global write "总磷总氮断电保存全局变量.vi" "简易流程路径"("简易流程路径") -> ()
                n173 = global write "总磷总氮断电保存全局变量.vi" "IP"("IP") -> ()
                n174 = global write "总磷总氮断电保存全局变量.vi" "盐度自动补偿："(w222) -> ()
                n175 = global write "总磷总氮断电保存全局变量.vi" "流程路径"("测试流程路径") -> ()
                n176 = global write "总磷总氮断电保存全局变量.vi" "标样核查自动补测"("标样核查自动补测") -> ()
                n177 = global write "总磷总氮断电保存全局变量.vi" "PORT"("PORT") -> ()
                n178 = global write "总磷总氮断电保存全局变量.vi" "跨度核查自动补测"("跨度核查自动补测") -> ()
                n179 = global write "总磷总氮断电保存全局变量.vi" "VISA Resource"("请选择串口:") -> ()
                n180 = global write "总磷总氮断电保存全局变量.vi" "零点核查自动补测"("零点核查自动补测") -> ()
                n181 = To Unsigned Word Integer(number=w224) -> (unsigned 16bit integer=w223:cluster{u16, u16, u16, u16, u16})
                n182 = global read "总磷总氮断电保存全局变量.vi" "低量程上限"() -> (w215:T15)
                n183 = property on="低量程上限" class="DigNum (严格)"() -> ("Value"=w213:dbl)  [unwired: 2 in, 2 out]
                n184 = global read "总磷总氮断电保存全局变量.vi" "质控参数设置"() -> (w230:T16)
                n185 = local read "消解时长"() -> (w217:dbl)
                n186 = case shown="1" w235 {
                  tunnel: "跨度值" -> [_ w250 w264 w277 w290 w303 w316 w329 w342 w356 w370 w383]
                  tunnel: "标样核查标液浓度" -> [_ w247 w261 w274 w287 w300 w313 w326 w339 w353 w367 w380]
                  tunnel: "跨度核查标液浓度" -> [_ w248 w262 w275 w288 w301 w314 w327 w340 w354 w368 w381]
                  tunnel: "零点核查标液浓度" -> [_ w249 w263 w276 w289 w302 w315 w328 w341 w355 w369 w382]
                  tunnel: w230 -> [_ w252 w266 w279 w292 w305 w318 w331 w344 w358 w372 w385]
                  tunnel: w223 -> [_ w246 w260 w273 w286 w299 w312 w325 w338 w351 w365 w379]
                  tunnel: w217 -> [_ w245 w259 _ _ _ _ _ _ w352 w366 _]
                  tunnel: w215 -> [w238 w243 w258 w272 w285 w298 w311 w324 w337 w350 w364 w378]
                  tunnel: [w238 w242 w256 w271 w284 w297 w310 w323 w336 w349 w363 w377] -> w214
                  tunnel: w213 -> [_ w244 w257 w270 w283 w296 w309 w322 w335 w348 w362 w376]
                  tunnel: "标样核查标液偏差" -> [_ w241 w253 w267 w280 w295 w306 w319 w332 w345 w359 w373]
                  tunnel: "跨度核查标液偏差" -> [_ w240 w254 w268 w281 w294 w307 w320 w333 w346 w360 w374]
                  tunnel: "零点核查标液偏差" -> [_ w239 w255 w269 w282 w293 w308 w321 w334 w347 w361 w375]
                  frame 0, Default {
                  }
                  frame 1 {
                    n187 = global write "总磷总氮断电保存全局变量.vi" "总磷自动测试量程配置"(w246) -> ()
                    n188 = global write "总磷总氮断电保存全局变量.vi" "总磷消解时长"(w245) -> ()
                    n189 = Bundle By Name(cluster=w243, "总磷"=w244) -> (w242:T15)
                    n190 = Bundle By Name(cluster=w252, "总磷跨度值"=w250, "总磷零点标准液浓度"=w249, "总磷跨度标准液浓度"=w248, "总磷标准液标准浓度"=w247, "总磷零点标准液偏差"=w239, "总磷跨度标准液偏差"=w240, "总磷标准液标准偏差"=w241) -> (w251:T16)
                    n191 = global write "总磷总氮断电保存全局变量.vi" "质控参数设置"(w251) -> ()
                  }
                  frame 2 {
                    n192 = global write "总磷总氮断电保存全局变量.vi" "总氮自动测试量程配置"(w260) -> ()
                    n193 = global write "总磷总氮断电保存全局变量.vi" "总氮消解时长"(w259) -> ()
                    n194 = Bundle By Name(cluster=w258, "总氮"=w257) -> (w256:T15)
                    n195 = Bundle By Name(cluster=w266, "总氮跨度值"=w264, "总氮零点标准液浓度"=w263, "总氮跨度标准液浓度"=w262, "总氮标准液标准浓度"=w261, "总氮零点标准液偏差"=w255, "总氮跨度标准液偏差"=w254, "总氮标准液标准偏差"=w253) -> (w265:T16)
                    n196 = global write "总磷总氮断电保存全局变量.vi" "质控参数设置"(w265) -> ()
                  }
                  frame 3 {
                    n197 = global write "总磷总氮断电保存全局变量.vi" "氨氮自动测试量程配置"(w273) -> ()
                    n198 = Bundle By Name(cluster=w272, "氨氮"=w270) -> (w271:T15)
                    n199 = Bundle By Name(cluster=w279, "氨氮跨度值"=w277, "氨氮零点标准液浓度"=w276, "氨氮跨度标准液浓度"=w275, "氨氮标准液标准浓度"=w274, "氨氮零点标准液偏差"=w269, "氨氮跨度标准液偏差"=w268, "氨氮标准液标准偏差"=w267) -> (w278:T16)
                    n200 = global write "总磷总氮断电保存全局变量.vi" "质控参数设置"(w278) -> ()
                  }
                  frame 4 {
                    n201 = global write "总磷总氮断电保存全局变量.vi" "磷酸盐自动测试量程配置"(w286) -> ()
                    n202 = Bundle By Name(cluster=w285, "磷酸盐"=w283) -> (w284:T15)
                    n203 = Bundle By Name(cluster=w292, "磷酸盐跨度值"=w290, "磷酸盐零点标准液浓度"=w289, "磷酸盐跨度标准液浓度"=w288, "磷酸盐标准液标准浓度"=w287, "磷酸盐零点标准液偏差"=w282, "磷酸盐跨度标准液偏差"=w281, "磷酸盐标准液标准偏差"=w280) -> (w291:T16)
                    n204 = global write "总磷总氮断电保存全局变量.vi" "质控参数设置"(w291) -> ()
                  }
                  frame 5 {
                    n205 = global write "总磷总氮断电保存全局变量.vi" "硝氮自动测试量程配置"(w299) -> ()
                    n206 = Bundle By Name(cluster=w298, "硝氮"=w296) -> (w297:T15)
                    n207 = Bundle By Name(cluster=w305, "硝氮跨度值"=w303, "硝氮零点标准液浓度"=w302, "硝氮跨度标准液浓度"=w301, "硝氮标准液标准浓度"=w300, "硝氮零点标准液偏差"=w293, "硝氮跨度标准液偏差"=w294, "硝氮标准液标准偏差"=w295) -> (w304:T16)
                    n208 = global write "总磷总氮断电保存全局变量.vi" "质控参数设置"(w304) -> ()
                  }
                  frame 6 {
                    n209 = global write "总磷总氮断电保存全局变量.vi" "亚硝氮自动测试量程配置"(w312) -> ()
                    n210 = Bundle By Name(cluster=w311, "亚硝氮"=w309) -> (w310:T15)
                    n211 = Bundle By Name(cluster=w318, "亚硝氮跨度值"=w316, "亚硝氮零点标准液浓度"=w315, "亚硝氮跨度标准液浓度"=w314, "亚硝氮标准液标准浓度"=w313, "亚硝氮零点标准液偏差"=w308, "亚硝氮跨度标准液偏差"=w307, "亚硝氮标准液标准偏差"=w306) -> (w317:T16)
                    n212 = global write "总磷总氮断电保存全局变量.vi" "质控参数设置"(w317) -> ()
                  }
                  frame 7 {
                    n213 = global write "总磷总氮断电保存全局变量.vi" "硅酸盐自动测试量程配置"(w325) -> ()
                    n214 = Bundle By Name(cluster=w324, "硅酸盐"=w322) -> (w323:T15)
                    n215 = Bundle By Name(cluster=w331, "硅酸盐跨度值"=w329, "硅酸盐零点标准液浓度"=w328, "硅酸盐跨度标准液浓度"=w327, "硅酸盐标准液标准浓度"=w326, "硅酸盐零点标准液偏差"=w321, "硅酸盐跨度标准液偏差"=w320, "硅酸盐标准液标准偏差"=w319) -> (w330:T16)
                    n216 = global write "总磷总氮断电保存全局变量.vi" "质控参数设置"(w330) -> ()
                  }
                  frame 8 {
                    n217 = global write "总磷总氮断电保存全局变量.vi" "硫化物自动测试量程配置"(w338) -> ()
                    n218 = Bundle By Name(cluster=w337, "硫化物"=w335) -> (w336:T15)
                    n219 = Bundle By Name(cluster=w344, "硫化物跨度值"=w342, "硫化物零点标准液浓度"=w341, "硫化物跨度标准液浓度"=w340, "硫化物标准液标准浓度"=w339, "硫化物零点标准液偏差"=w334, "硫化物跨度标准液偏差"=w333, "硫化物标准液标准偏差"=w332) -> (w343:T16)
                    n220 = global write "总磷总氮断电保存全局变量.vi" "质控参数设置"(w343) -> ()
                  }
                  frame 22 {
                    n221 = global write "总磷总氮断电保存全局变量.vi" "COD自动测试量程配置"(w351) -> ()
                    n222 = global write "总磷总氮断电保存全局变量.vi" "CODcr消解时长"(w352) -> ()
                    n223 = Bundle By Name(cluster=w350, "COD"=w348) -> (w349:T15)
                    n224 = Bundle By Name(cluster=w358, "COD跨度值"=w356, "COD零点标准液浓度"=w355, "COD跨度标准液浓度"=w354, "COD标准液标准浓度"=w353, "COD零点标准液偏差"=w347, "COD跨度标准液偏差"=w346, "COD标准液标准偏差"=w345) -> (w357:T16)
                    n225 = global write "总磷总氮断电保存全局变量.vi" "质控参数设置"(w357) -> ()
                  }
                  frame 21 {
                    n226 = global write "总磷总氮断电保存全局变量.vi" "CODMn自动测试量程配置"(w365) -> ()
                    n227 = global write "总磷总氮断电保存全局变量.vi" "CODmn消解时长"(w366) -> ()
                    n228 = Bundle By Name(cluster=w364, "CODMn"=w362) -> (w363:T15)
                    n229 = Bundle By Name(cluster=w372, "CODMn跨度值"=w370, "CODMn零点标准液浓度"=w369, "CODMn跨度标准液浓度"=w368, "CODMn标准液标准浓度"=w367, "CODMn零点标准液偏差"=w361, "CODMn跨度标准液偏差"=w360, "CODMn标准液标准偏差"=w359) -> (w371:T16)
                    n230 = global write "总磷总氮断电保存全局变量.vi" "质控参数设置"(w371) -> ()
                  }
                  frame 50 {
                    n231 = global write "总磷总氮断电保存全局变量.vi" "氟化物自动测试量程配置"(w379) -> ()
                    n232 = Bundle By Name(cluster=w378, "氟化物"=w376) -> (w377:T15)
                    n233 = Bundle By Name(cluster=w385, "氟化物跨度值"=w383, "氟化物零点标准液浓度"=w382, "氟化物跨度标准液浓度"=w381, "氟化物标准液标准浓度"=w380, "氟化物零点标准液偏差"=w375, "氟化物跨度标准液偏差"=w374, "氟化物标准液标准偏差"=w373) -> (w384:T16)
                    n234 = global write "总磷总氮断电保存全局变量.vi" "质控参数设置"(w384) -> ()
                  }
                }
                n235 = global write "总磷总氮断电保存全局变量.vi" "低量程上限"(w214) -> ()
              }
              frame #1 {
                n236 = Get Date/Time In Seconds() -> (seconds since 1Jan1904=w388:timestamp)
                n237 = property on="参数下拉列表" class="Ring (严格)"() -> ("RingText.Text"=w386:string)  [unwired: 2 in, 2 out]
                n238 = Bundle By Name(cluster=T8 {"时间"=timestamp(0 s since 1904-01-01), "参数"="", "日志信息"="", "流程参数"=""} ("data in"), "时间"=w388, "参数"=w386, "日志信息"="参数变更") -> (w389:T8)
                n239 = call "总磷总氮操作日志.vi"("data in"=w389) -> ()  [unwired: 10 in, 1 out]
                n240 = call "仪器配置写入.vi"() -> ()  [unwired: 11 in, 1 out]
              }
            }
          }
        }
      }
      event "通讯连接": Value Change {
        n241 = event-data() -> ("NewVal"=w391:bool)  [unwired: 1 in, 5 out]
        n242 = Flush Queue(queue=w392) -> (queue out=w393:refnum<queue>)  [unwired: 1 in, 2 out]
        n243 = case shown="假" w391 {
          tunnel: w393 -> [w394 w396]
          frame False {
            n244 = Enqueue Element At Opposite End(queue=w394, element=cluster{"命令":string, "data":variant} {"命令"="停用模块", "data"=variant} ("元素")) -> ()  [unwired: 2 in, 3 out]
          }
          frame True {
            n245 = Enqueue Element At Opposite End(queue=w396, element=cluster{"命令":string, "data":variant} {"命令"="启用模块", "data"=variant} ("元素")) -> ()  [unwired: 2 in, 3 out]
          }
        }
      }
      event "手动模式": Value Change {
        n246 = event-data() -> ()  [unwired: 1 in, 6 out]
        n247 = global write "VAR总磷总氮全局变量.vi" "手动模式"("手动模式") -> ()
      }
    }
  }
  n248 = while {
    tunnel: w7 -> [w409]
    tunnel: w8 -> [w408]
    tunnel: w9 -> [w407]
    tunnel: w6 -> [w406]
    stop <- FALSE stop-if-true
    n249 = Wait on Occurrence(2:w406) -> (0:w400:bool)  [unwired: 2 in]
    n250 = flat-sequence {
      tunnel: w409 -> [w416]
      tunnel: w408 -> [w415]
      tunnel: w407 -> [w414]
      tunnel: [w413] -> w403
      tunnel: [w412] -> w402
      tunnel: [w411] -> w401
      tunnel: w400 -> [_]
      frame #0 {
        n251 = property class="Enum (严格)"(reference=w415) -> ("Value"=w412:enum16{"低量程", "高量程"})  [unwired: 1 in, 2 out]
        n252 = property class="Ring (严格)"(reference=w416) -> ("Value"=w413:u16)  [unwired: 1 in, 2 out]
        n253 = property class="Enum (严格)"(reference=w414) -> ("Value"=w411:T1)  [unwired: 1 in, 2 out]
      }
    }
    n254 = flat-sequence {
      tunnel: [w419] -> w405
      tunnel: [w418] -> w404
      tunnel: w403 -> [w417]
      tunnel: w402 -> [w419]
      tunnel: w401 -> [w418]
      tunnel: [w417] -> w399
      tunnel: w405 -> [w438]
      tunnel: w404 -> [w439]
      tunnel: w399 -> [w437]
      frame #0 {
      }
      frame #1 {
        n255 = call "量程参数读取.vi"("测量参数"=w437) -> ("error out"=w428:errorcluster, "量程参数读取"=w436:T7)  [unwired: 9 in]
        n256 = Unbundle By Name(w436) -> ("测量精度"=→"测量精度":u16, "检出限"=→"检出限":dbl, "上限"=→"高量程上限":dbl, "下限"=→"量程下限":dbl, "阈值（低->高）"=→"阈值（低->高）":dbl, "阈值（高->低）"=→"阈值（高->低）":dbl, "稀释度"=→"稀释度":dbl)
        n257 = call "公式读取.vi"("error in (no error)"=w428, "量程"=w438, "测量模式"=w439, "测量参数"=w437) -> ("error out"=w422:errorcluster, "公式"=w427:cluster{"X^2":dbl, "X":dbl, "b":dbl})  [unwired: 6 in]
        n258 = Unbundle By Name(w427) -> ("X^2"=→"二次多项式系数":dbl, "X"=→"曲线斜率":dbl, "b"=→"曲线截距":dbl)
        n259 = global read "VAR总磷总氮全局变量.vi" "MB session in"() -> (w421:refnum<class "MB_Master.lvclass">)
        n260 = case shown="1, 2, 21, 22" w437 {
          tunnel: [_ w442] -> w423
          tunnel: [w440 w448] -> _
          tunnel: w422 -> [w440 w443]
          tunnel: w421 -> [_ w446]
          tunnel: [_ w447] -> w420
          frame 0, Default {
          }
          frame 1, 2, 21, 22 {
            n261 = call "版本判断.vi"() -> ("仪器版本"=w445:T9)  [unwired: 11 in]
            n262 = case shown="\"V4.2版\"" w445 {
              tunnel: [w454 w458 w463 w469] -> w444
              tunnel: w446 -> [w453 w459 w464 w470]
              tunnel: [w450 w456 w461 w467] -> w442
              tunnel: w443 -> [w452 _ _ w466]
              tunnel: [w449 w455 w460 w465] -> w441
              frame "V3.1版", Default {
                n263 = call "读取V3.1外设配置.vi"("error in (no error)"=w452, "MB session in"=w453) -> ("error out"=w454:errorcluster, "外设配置"=w451:T10, "MB session out"=w449:refnum<class "MB_Master.lvclass">)  [unwired: 7 in]
                n264 = Unbundle By Name(w451) -> ("消解温度下限"=w450:sgl)
              }
              frame "V4版" {
                n265 = call "读取V4版外设配置.vi"("MB session in"=w459) -> ("error out"=w458:errorcluster, "外设配置"=w457:T11, "MB session out"=w455:refnum<class "MB_Master.lvclass">)  [unwired: 8 in]
                n266 = Unbundle By Name(w457) -> ("消解温度下限"=w456:sgl)
              }
              frame "V4.2版" {
                n267 = call "读取V4.2版外设配置.vi"("MB session in"=w464) -> ("error out"=w463:errorcluster, "外设配置"=w462:T12, "MB session out"=w460:refnum<class "MB_Master.lvclass">)  [unwired: 8 in]
                n268 = Unbundle By Name(w462) -> ("消解温度"=w461:sgl)
              }
              frame "V3版" {
                n269 = call "读取V3外设配置.vi"("error in (no error)"=w466, "MB session in"=w470) -> ("error out"=w469:errorcluster, "外设配置"=w468:T13, "MB session out"=w465:refnum<class "MB_Master.lvclass">)  [unwired: 7 in]
                n270 = Unbundle By Name(w468) -> ("消解温度下限"=w467:sgl)
              }
            }
            n271 = call "盐度补偿值读取.vi"("Error in"=w444, "MB session in"=w441) -> ("error out"=w448:errorcluster, "盐度补偿值"=w447:sgl)  [unwired: 7 in, 1 out]
          }
        }
        "消解温度" <- w423
        "盐度补偿值" <- w420
      }
      frame #2 {
        n272 = Format Date/Time String() -> (date/time string=→"数据刷新时间":string)  [unwired: 3 in]
      }
    }
  }
  n273 = while {
    tunnel: w7 -> [w482]
    stop <- FALSE stop-if-true
    n274 = global read "总磷总氮断电保存全局变量.vi" "盐度自动补偿："() -> (w497:bool)
    n275 = property class="Ring (严格)"(reference=w482) -> ("Value"=w481:u16)  [unwired: 1 in, 2 out]
    n276 = global read "总磷总氮断电保存全局变量.vi" "跨度核查自动补测"() -> (w472:bool)
    n277 = global read "总磷总氮断电保存全局变量.vi" "MB通信方式选择"() -> (w496:enum16{"串口", "TCP"})
    n278 = global read "总磷总氮断电保存全局变量.vi" "VISA Resource"() -> (w501:refnum<visa-resource-name>)
    n279 = global read "总磷总氮断电保存全局变量.vi" "简易流程路径"() -> (w480:path)
    n280 = global read "总磷总氮断电保存全局变量.vi" "零点核查自动补测"() -> (w474:bool)
    n281 = global read "总磷总氮断电保存全局变量.vi" "标样核查自动补测"() -> (w473:bool)
    n282 = global read "总磷总氮断电保存全局变量.vi" "流程路径"() -> (w498:path)
    n283 = global read "总磷总氮断电保存全局变量.vi" "PORT"() -> (w500:string)
    n284 = local write "盐度自动补偿："(w497) -> ()
    n285 = global read "总磷总氮断电保存全局变量.vi" "质控参数设置"() -> (w491:T16)
    n286 = global read "总磷总氮断电保存全局变量.vi" "低量程上限"() -> (w479:T15)
    n287 = local write "跨度核查自动补测"(w472) -> ()
    n288 = local write "通信方式选择"(w496) -> ()
    n289 = local write "请选择串口:"(w501) -> ()
    n290 = local write "简易流程路径"(w480) -> ()
    n291 = local write "零点核查自动补测"(w474) -> ()
    n292 = local write "标样核查自动补测"(w473) -> ()
    n293 = local write "测试流程路径"(w498) -> ()
    n294 = local write "PORT"(w500) -> ()
    n295 = case shown="21" w481 {
      tunnel: [_ w516 w528 w539 w550 w561 w572 w583 w594 w606 w617 w629] -> w489
      tunnel: [_ w515 w527 _ _ _ _ _ _ w605 _ w618] -> w490
      tunnel: w491 -> [_ w514 w526 w538 w549 w560 w571 w582 w593 w604 w616 w628]
      tunnel: [_ w513 w525 w537 w548 w559 w570 w581 w592 w603 w615 w627] -> w492
      tunnel: [_ w512 w524 w536 w547 w558 w569 w580 w591 w602 w614 w626] -> w493
      tunnel: [_ w511 w523 w535 w546 w557 w568 w579 w590 w601 w613 w625] -> w494
      tunnel: [_ w510 w522 w534 w545 w556 w567 w578 w589 w600 w612 w624] -> w495
      tunnel: w479 -> [_ w509 w521 w533 w544 w555 w566 w577 w588 w599 w611 w623]
      tunnel: [0.0 ("COD") w508 w520 w532 w543 w554 w565 w576 w587 w598 w610 w622] -> w478
      tunnel: [_ w507 w519 w531 w542 w553 w564 w575 w586 w597 w609 w621] -> w477
      tunnel: [_ w506 w518 w530 w541 w552 w563 w574 w585 w596 w608 w620] -> w476
      tunnel: [_ w505 w517 w529 w540 w551 w562 w573 w584 w595 w607 w619] -> w475
      frame Default {
      }
      frame 1 {
        n296 = Unbundle By Name(w514) -> ("总磷跨度值"=w513:dbl, "总磷零点标准液浓度"=w512:dbl, "总磷跨度标准液浓度"=w511:dbl, "总磷标准液标准浓度"=w510:dbl, "总磷零点标准液偏差"=w507:dbl, "总磷跨度标准液偏差"=w506:dbl, "总磷标准液标准偏差"=w505:dbl)
        n297 = Unbundle By Name(w509) -> ("总磷"=w508:dbl)
        n298 = global read "总磷总氮断电保存全局变量.vi" "总磷消解时长"() -> (w515:dbl)
        n299 = global read "总磷总氮断电保存全局变量.vi" "总磷自动测试量程配置"() -> (w516:T17)
      }
      frame 2 {
        n300 = Unbundle By Name(w526) -> ("总氮跨度值"=w525:dbl, "总氮零点标准液浓度"=w524:dbl, "总氮跨度标准液浓度"=w523:dbl, "总氮标准液标准浓度"=w522:dbl, "总氮零点标准液偏差"=w519:dbl, "总氮跨度标准液偏差"=w518:dbl, "总氮标准液标准偏差"=w517:dbl)
        n301 = Unbundle By Name(w521) -> ("总氮"=w520:dbl)
        n302 = global read "总磷总氮断电保存全局变量.vi" "总氮消解时长"() -> (w527:dbl)
        n303 = global read "总磷总氮断电保存全局变量.vi" "总氮自动测试量程配置"() -> (w528:T17)
      }
      frame 3 {
        n304 = Unbundle By Name(w538) -> ("氨氮跨度值"=w537:dbl, "氨氮零点标准液浓度"=w536:dbl, "氨氮跨度标准液浓度"=w535:dbl, "氨氮标准液标准浓度"=w534:dbl, "氨氮零点标准液偏差"=w531:dbl, "氨氮跨度标准液偏差"=w530:dbl, "氨氮标准液标准偏差"=w529:dbl)
        n305 = Unbundle By Name(w533) -> ("氨氮"=w532:dbl)
        n306 = global read "总磷总氮断电保存全局变量.vi" "氨氮自动测试量程配置"() -> (w539:T17)
      }
      frame 4 {
        n307 = Unbundle By Name(w549) -> ("磷酸盐跨度值"=w548:dbl, "磷酸盐零点标准液浓度"=w547:dbl, "磷酸盐跨度标准液浓度"=w546:dbl, "磷酸盐标准液标准浓度"=w545:dbl, "磷酸盐零点标准液偏差"=w542:dbl, "磷酸盐跨度标准液偏差"=w541:dbl, "磷酸盐标准液标准偏差"=w540:dbl)
        n308 = Unbundle By Name(w544) -> ("磷酸盐"=w543:dbl)
        n309 = global read "总磷总氮断电保存全局变量.vi" "磷酸盐自动测试量程配置"() -> (w550:T17)
      }
      frame 5 {
        n310 = Unbundle By Name(w560) -> ("硝氮跨度值"=w559:dbl, "硝氮零点标准液浓度"=w558:dbl, "硝氮跨度标准液浓度"=w557:dbl, "硝氮标准液标准浓度"=w556:dbl, "硝氮零点标准液偏差"=w553:dbl, "硝氮跨度标准液偏差"=w552:dbl, "硝氮标准液标准偏差"=w551:dbl)
        n311 = Unbundle By Name(w555) -> ("硝氮"=w554:dbl)
        n312 = global read "总磷总氮断电保存全局变量.vi" "硝氮自动测试量程配置"() -> (w561:T17)
      }
      frame 6 {
        n313 = Unbundle By Name(w571) -> ("亚硝氮跨度值"=w570:dbl, "亚硝氮零点标准液浓度"=w569:dbl, "亚硝氮跨度标准液浓度"=w568:dbl, "亚硝氮标准液标准浓度"=w567:dbl, "亚硝氮零点标准液偏差"=w564:dbl, "亚硝氮跨度标准液偏差"=w563:dbl, "亚硝氮标准液标准偏差"=w562:dbl)
        n314 = Unbundle By Name(w566) -> ("亚硝氮"=w565:dbl)
        n315 = global read "总磷总氮断电保存全局变量.vi" "亚硝氮自动测试量程配置"() -> (w572:T17)
      }
      frame 7 {
        n316 = Unbundle By Name(w582) -> ("硅酸盐跨度值"=w581:dbl, "硅酸盐零点标准液浓度"=w580:dbl, "硅酸盐跨度标准液浓度"=w579:dbl, "硅酸盐标准液标准浓度"=w578:dbl, "硅酸盐零点标准液偏差"=w575:dbl, "硅酸盐跨度标准液偏差"=w574:dbl, "硅酸盐标准液标准偏差"=w573:dbl)
        n317 = Unbundle By Name(w577) -> ("硅酸盐"=w576:dbl)
        n318 = global read "总磷总氮断电保存全局变量.vi" "硅酸盐自动测试量程配置"() -> (w583:T17)
      }
      frame 8 {
        n319 = Unbundle By Name(w593) -> ("硫化物跨度值"=w592:dbl, "硫化物零点标准液浓度"=w591:dbl, "硫化物跨度标准液浓度"=w590:dbl, "硫化物标准液标准浓度"=w589:dbl, "硫化物零点标准液偏差"=w586:dbl, "硫化物跨度标准液偏差"=w585:dbl, "硫化物标准液标准偏差"=w584:dbl)
        n320 = Unbundle By Name(w588) -> ("硫化物"=w587:dbl)
        n321 = global read "总磷总氮断电保存全局变量.vi" "硫化物自动测试量程配置"() -> (w594:T17)
      }
      frame 22 {
        n322 = Unbundle By Name(w604) -> ("COD跨度值"=w603:dbl, "COD零点标准液浓度"=w602:dbl, "COD跨度标准液浓度"=w601:dbl, "COD标准液标准浓度"=w600:dbl, "COD零点标准液偏差"=w597:dbl, "COD跨度标准液偏差"=w596:dbl, "COD标准液标准偏差"=w595:dbl)
        n323 = Unbundle By Name(w599) -> ("COD"=w598:dbl)
        n324 = global read "总磷总氮断电保存全局变量.vi" "CODcr消解时长"() -> (w605:dbl)
        n325 = global read "总磷总氮断电保存全局变量.vi" "COD自动测试量程配置"() -> (w606:T17)
      }
      frame 50 {
        n326 = Unbundle By Name(w616) -> ("氟化物跨度值"=w615:dbl, "氟化物零点标准液浓度"=w614:dbl, "氟化物跨度标准液浓度"=w613:dbl, "氟化物标准液标准浓度"=w612:dbl, "氟化物零点标准液偏差"=w609:dbl, "氟化物跨度标准液偏差"=w608:dbl, "氟化物标准液标准偏差"=w607:dbl)
        n327 = Unbundle By Name(w611) -> ("氟化物"=w610:dbl)
        n328 = global read "总磷总氮断电保存全局变量.vi" "氟化物自动测试量程配置"() -> (w617:T17)
      }
      frame 21 {
        n329 = Unbundle By Name(w628) -> ("CODMn跨度值"=w627:dbl, "CODMn零点标准液浓度"=w626:dbl, "CODMn跨度标准液浓度"=w625:dbl, "CODMn标准液标准浓度"=w624:dbl, "CODMn零点标准液偏差"=w621:dbl, "CODMn跨度标准液偏差"=w620:dbl, "CODMn标准液标准偏差"=w619:dbl)
        n330 = Unbundle By Name(w623) -> ("CODMn"=w622:dbl)
        n331 = global read "总磷总氮断电保存全局变量.vi" "CODMn自动测试量程配置"() -> (w629:T17)
        n332 = global read "总磷总氮断电保存全局变量.vi" "CODcr消解时长"() -> (w618:dbl)
      }
    }
    "消解时长" <- w490
    "低量程上限" <- w478
    n333 = global read "总磷总氮断电保存全局变量.vi" "IP"() -> (w499:string)
    n334 = local write "IP"(w499) -> ()
    n335 = Wait (ms)(milliseconds to wait=u32 1000 ("等待时间（毫秒）")) -> ()  [unwired: 1 out]
    n336 = local write "跨度值"(w492) -> ()
    n337 = local write "零点核查标液浓度"(w493) -> ()
    n338 = local write "跨度核查标液浓度"(w494) -> ()
    n339 = local write "标样核查标液浓度"(w495) -> ()
    n340 = local write "零点核查标液偏差"(w477) -> ()
    n341 = local write "跨度核查标液偏差"(w476) -> ()
    n342 = local write "标样核查标液偏差"(w475) -> ()
    n343 = To Unsigned Word Integer(number=w489) -> (unsigned 16bit integer=w488:T18)
    n344 = Unbundle By Name(w488) -> ("水样测试量程模式"=w487:u16, "空白核查量程模式"=w485:u16, "跨度核查量程模式"=w484:u16, "加标回收量程模式"=w483:u16, "标样核查量程模式"=w486:u16)
    n345 = local write "水样测试量程模式"(w487) -> ()
    n346 = local write "零点核查量程模式"(w485) -> ()
    n347 = local write "跨度核查量程模式"(w484) -> ()
    n348 = local write "加标回收量程模式"(w483) -> ()
    n349 = local write "标样核查量程模式"(w486) -> ()
  }
